vi "SI100.vi"(0 "Redundance":enum16{"10", "20", "30", "40"}(ring), 1 "APs":cluster{"AP1":dbl, "AP2":dbl, "AP3":dbl}, 2 "3 JEC CT953 XQ01":dbl, 3 "3 JEC CT951 XQ01":dbl, 4 "3 JEC CT953 XQ01":dbl, 5 "3 JEC CT952 XQ01":dbl) -> (14 "Avg Temp Rise":dbl, 15 "T-Rise 2nd Max":dbl, 17 "Aps out":cluster{"AP1":dbl, "AP2":dbl, "AP3":dbl})   [LabVIEW 2022 SP3, in "SI100_ReactorTemperatureRise.lvclass"]
uses:
  SI100_ReactorTemperatureRise.lvclass
  b0afb3a3-63e2-41d1-9697-9d4c6fa37d5c.vi
  <vilib>/Comparison/Less/Less Functor/Less Functor.lvclass
  SIClass/SIClass.lvclass
  SI100_ReactorTemperatureRise.lvclass/SI100_ReactorTemperatureRise.ctl
panel:
  in  "error in":errorcluster
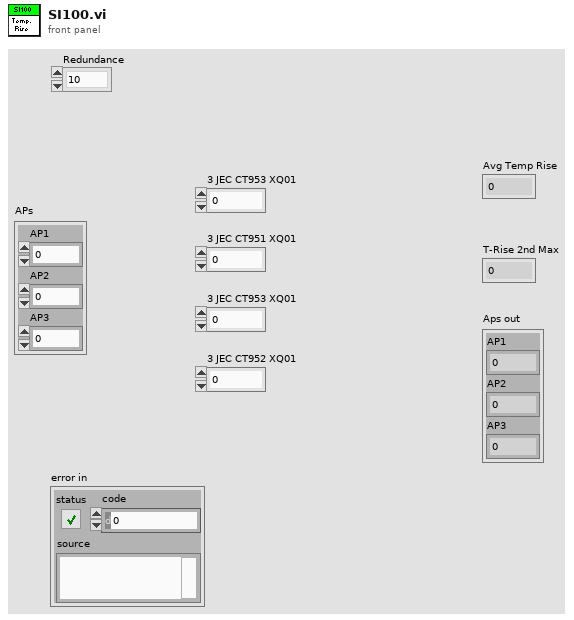
[diagram p1: front panel]
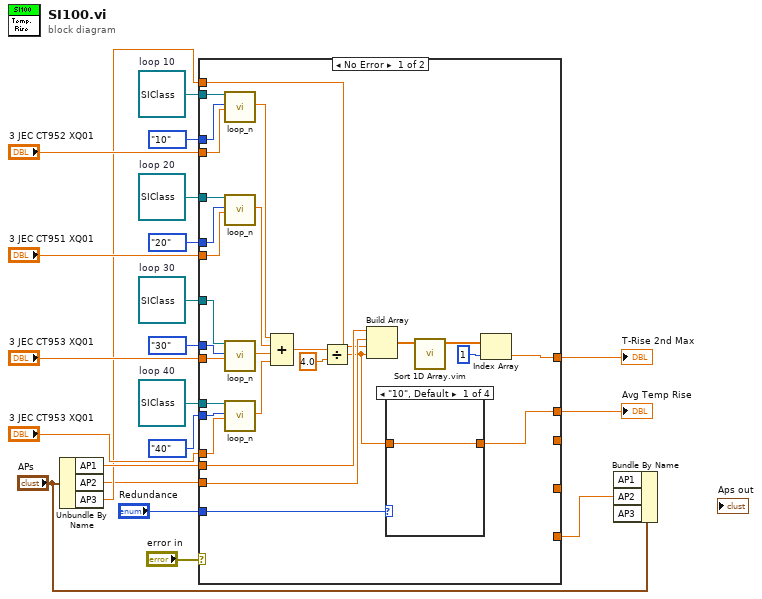
[diagram p0: block diagram]
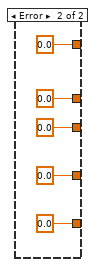
[diagram p5: hidden frame]
diagram:
  w10 = refnum<class "SIClass.lvclass"> refnum  # loop 40
  w13 = refnum<class "SIClass.lvclass"> refnum  # loop 30
  w18 = refnum<class "SIClass.lvclass"> refnum  # loop 20
  w21 = refnum<class "SIClass.lvclass"> refnum  # loop 10
  n1 = Unbundle By Name("APs") -> ("AP1"=w6:dbl, "AP2"=w4:dbl, "AP3"=w5:dbl)
  n2 = case shown="No Error" "error in" {
    tunnel: w21 -> [w49 _]
    tunnel: enum16{"10", "20", "30", "40"}."10" ("Loop ID") -> [w48 _]
    tunnel: "3 JEC CT952 XQ01" -> [w47 _]
    tunnel: w18 -> [w46 _]
    tunnel: enum16{"10", "20", "30", "40"}."20" ("Loop ID 2") -> [w45 _]
    tunnel: "3 JEC CT951 XQ01" -> [w44 _]
    tunnel: "3 JEC CT953 XQ01" -> [w43 _]
    tunnel: enum16{"10", "20", "30", "40"}."30" ("Loop ID 3") -> [w42 _]
    tunnel: w13 -> [w41 _]
    tunnel: "3 JEC CT953 XQ01" -> [w40 _]
    tunnel: enum16{"10", "20", "30", "40"}."40" ("Loop ID 4") -> [w39 _]
    tunnel: w10 -> [w38 _]
    tunnel: [w25 0.0] -> w9
    tunnel: w6 -> [w27 _]
    tunnel: w4 -> [w26 _]
    tunnel: w5 -> [w24 _]
    tunnel: "Redundance" -> [w28 _]
    tunnel: [_ 0.0 ("AP1")] -> _
    tunnel: [_ 0.0 ("AP2")] -> w1
    tunnel: [_ 0.0 ("AP2")] -> _
    tunnel: [w22 0.0 ("AP2")] -> w2
    frame No Error {
      n3 = call-dynamic "loop_n.vi"("SIClass in"=w49, "Loop ID"=w48, "Input"=w47) -> ("Output"=w37:dbl)  [unwired: 14 in, 2 out]
      n4 = call-dynamic "loop_n.vi"("SIClass in"=w46, "Loop ID"=w45, "Input"=w44) -> ("Output"=w36:dbl)  [unwired: 14 in, 2 out]
      n5 = call-dynamic "loop_n.vi"("SIClass in"=w41, "Loop ID"=w42, "Input"=w43) -> ("Output"=w35:dbl)  [unwired: 14 in, 2 out]
      n6 = call-dynamic "loop_n.vi"("SIClass in"=w38, "Loop ID"=w39, "Input"=w40) -> ("Output"=w34:dbl)  [unwired: 14 in, 2 out]
      n7 = Compound Arithmetic op=ADD(w37, w36, w35, w34) -> (w33:dbl)
      n8 = Divide(x=w33, y=4.0) -> (x/y=w23:dbl)
      n9 = Build Array(w27, w26, w24, w23) -> (w31:dbl[])
      n10 = case shown="\"10\", Default" w28 {
        tunnel: w23 -> [w50 _ _ _]
        tunnel: [w50 _ _ _] -> w22
        frame "10", Default {
        }
        frame "20" {
          # "SI101"
        }
        frame "30" {
        }
        frame "40" {
          # "SI101"
        }
      }
      n11 = call "Sort 1D Array.vim"("unsorted array"=w31) -> ("sorted array"=w30:dbl[])  [unwired: 10 in]
      n12 = Index Array(array=w30, index=1) -> (element=w25:dbl)
    }
    frame Error {
    }
  }
  "T-Rise 2nd Max" <- w9
  "Avg Temp Rise" <- w2
  n13 = Bundle By Name(cluster="APs", "AP2"=w1) -> ()  [unwired: 2 in, 1 out]
